vi "Step Response (16 bit).vi"() -> ()   [LabVIEW 2012]
uses:
  Madlib.dll
panel:
  in  "Step size":dbl=25.0 min=0.0 max=100.0 format="%.2f"
  out "XY Graph 2":cluster{dbl[], "Data Array Out":dbl[]}(graph) caption="Step Response"
  in  "Axis":u32=1 min=1 max=3
  in  "ADC Rate (ms)":dbl=0.033333 min=0.03333 max=5.0 format="%.4f"
  in  "Number of Positions\nto Read":u32=1000 min=1 max=10000
  # "X = 1\nY = 2\nZ = 3"
  # "Percentage of the range of\nmotion to step.  Step will be\ncentered at 50% of the range\nof motion.  A step of 25% will \nmove the axis from 37.5% of\nits range of motion to 62.5%\nof its range of motion."
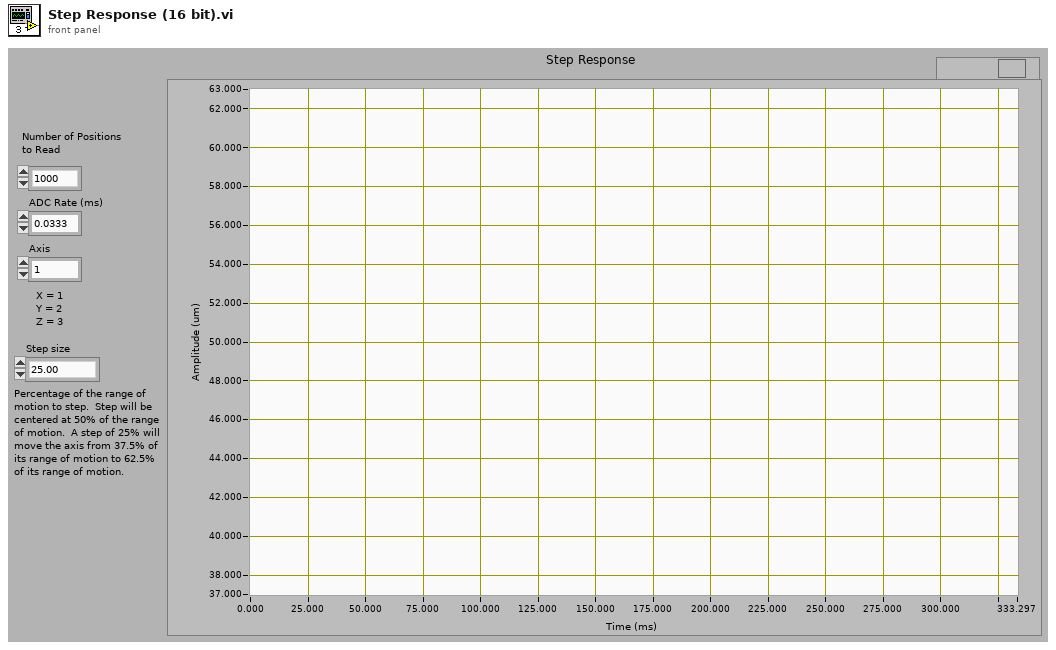
[diagram p1: front panel]
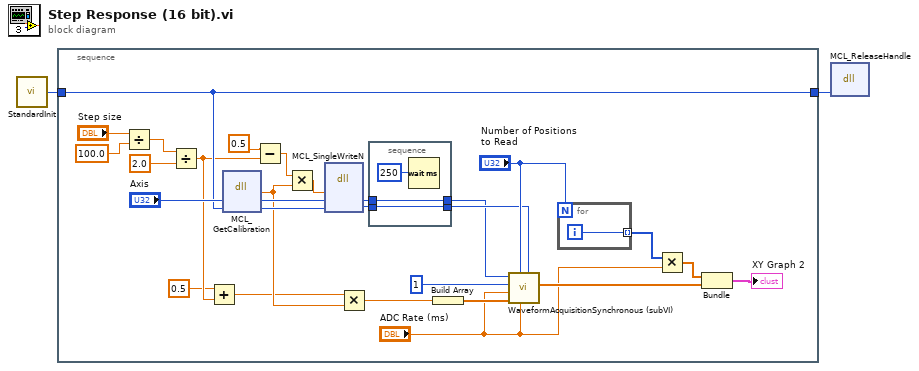
[diagram p0: block diagram]
diagram:
  n1 = call "StandardInit.vi"() -> ("Outgoing Handle"=w2:i32)  [unwired: 1 in]
  n2 = stacked-sequence {
    tunnel: w2 -> [w12]
    tunnel: [w12] -> w1
    frame #0 {
      n3 = Divide(x="Step size", y=100.0) -> (x/y=w3:dbl)
      n4 = Divide(x=w3, y=2.0) -> (x/y=w8:dbl)
      n5 = Add(x=0.5, y=w8) -> (x+y=w6:dbl)
      n6 = dll-call lib="C:/Users/Labview/Desktop/SRR/Madlib_x64/Labview Examples/MADLib.dll" fn="MCL_GetCalibration"("axis"="Axis", "handle"=w12) -> (w15:dbl, "axis"=w19:u32, "handle"=w20:i32)  [unwired: 3 in, 2 out]
      n7 = Subtract(x=0.5, y=w8) -> (x-y=w11:dbl)
      n8 = Multiply(x=w11, y=w15) -> (x*y=w14:dbl)
      n9 = dll-call lib="C:/Users/Labview/Desktop/SRR/Madlib_x64/Labview Examples/MADLib.dll" fn="MCL_SingleWriteN"("position"=w14, "axis"=w19, "handle"=w20) -> ("axis"=w18:u32, "handle"=w22:i32)  [unwired: 5 in, 2 out]
      n10 = Multiply(x=w6, y=w15) -> (x*y=w23:dbl)
      n11 = stacked-sequence {
        tunnel: [w32] -> w17
        tunnel: w22 -> [w32]
        tunnel: [w31] -> w16
        tunnel: w18 -> [w31]
        frame #0 {
          n12 = Wait (ms)(milliseconds to wait=250) -> ()  [unwired: 1 out]
        }
      }
      n13 = Build Array(w23) -> (w27:dbl[])
      n14 = call "WaveformAcquisitionSynchronous (subVI).vi"("Handle"=w17, "ADC Rate (ms)"="ADC Rate (ms)", "Number of Positions to Read"="Number of Positions\nto Read", "Data Array In"=w27, "DAC Rate (ms)"="ADC Rate (ms)", "Number of Steps"=1, "Axis"=w16) -> ("Data Array Out"=w24:dbl[])  [unwired: 2 in, 1 out]
      n15 = for {
        N: "Number of Positions\nto Read" -> [_]
        tunnel: [w34] -> w30 mode=indexing
        i -> [w34]
      }
      n16 = Multiply(x=w30, y="ADC Rate (ms)") -> (x*y=w29:dbl[])
      n17 = Bundle(w29, "Data Array Out"=w24) -> (→"XY Graph 2":cluster{dbl[], "Data Array Out":dbl[]})  [unwired: 1 in]
    }
  }
  n18 = dll-call lib="C:/Users/Labview/Desktop/SRR/Madlib_x64/Labview Examples/MADLib.dll" fn="MCL_ReleaseHandle"("handle"=w1) -> ()  [unwired: 5 in, 2 out]
